vi "Close DO Ref.vi"(8 "error in (no error)":errorcluster, 11 "PXI 6515 in":refnum<class "PXI 6515.lvclass">) -> (0 "error out":errorcluster, 3 "PXI 6515 out":refnum<class "PXI 6515.lvclass">)   [LabVIEW 2016, in "DAQ IO.lvlib" / "PXI 6515.lvclass"]
uses:
  PXI 6515.lvclass
  PXI 6515.lvclass/PXI 6515.ctl
  <vilib>/DAQmx/write.llb/DAQmx Write (Digital Bool 1Line 1Point).vi
  <vilib>/DAQmx/miscellaneous.llb/DAQmx Fill In Error Info.vi
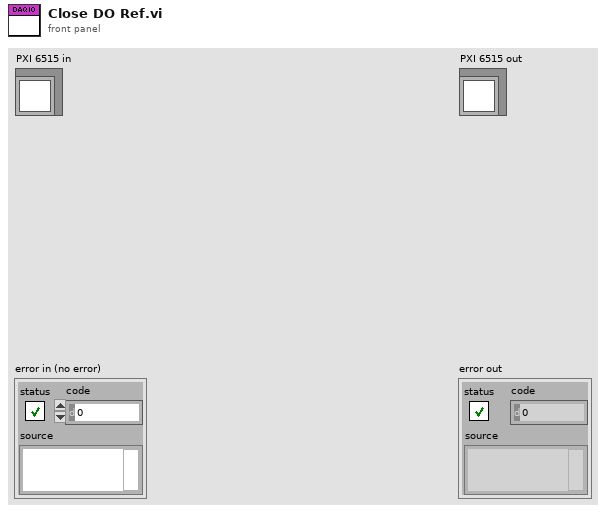
[diagram p1: front panel]
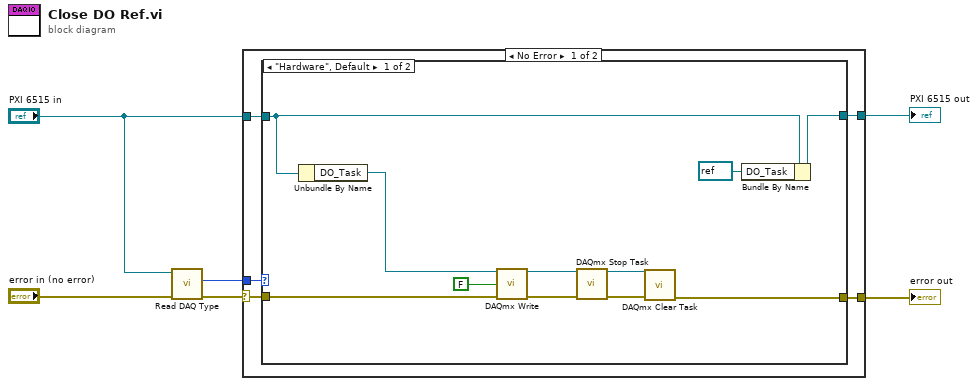
[diagram p0: block diagram]
diagram:
  n1 = call-dynamic "Read DAQ Type.vi"("error in (no error)"="error in (no error)", "PXI 6515 in"="PXI 6515 in") -> ("error out"=w5:errorcluster, "DAQ Type"=w4:enum16{"Hardware", "Simulation"})  [unwired: 7 in, 1 out]
  n2 = case shown="No Error" w5 {
    selector: w5 -> [w11 w25]
    tunnel: w4 -> [w10 _]
    tunnel: "PXI 6515 in" -> [w9 w26]
    tunnel: [w8 w25] -> w2
    tunnel: [w7 w26] -> w1
    frame No Error {
      n3 = case shown="\"Hardware\", Default" w10 {
        tunnel: w11 -> [w22 w23]
        tunnel: w9 -> [w20 w24]
        tunnel: [w21 w23] -> w8
        tunnel: [w19 w24] -> w7
        frame "Hardware", Default {
          n4 = Unbundle By Name(w20) -> ("DO_Task"=w13:refnum<k21>)
          n5 = call-poly <vilib>:"DAQmx Write.vi"("task/channels in"=w13, "data"=FALSE, "error in"=w22) -> ("task out"=w15:refnum<k21>, "error out"=w17:errorcluster)  [unwired: 10 in, 1 out]
          n6 = call <vilib>:"DAQmx Stop Task.vi"("task/channels in"=w15, "error in"=w17) -> ("task out"=w14:refnum<k21>, "error out"=w16:errorcluster)  [unwired: 12 in]
          n7 = call <vilib>:"DAQmx Clear Task.vi"("task in"=w14, "error in"=w16) -> ("error out"=w21:errorcluster)  [unwired: 13 in]
          n8 = Bundle By Name(cluster=w20, "DO_Task"=refnum<k21> refnum) -> (w19:refnum<class "PXI 6515.lvclass">)
        }
        frame "Simulation" {
        }
      }
    }
    frame Error {
    }
  }
  "error out" <- w2
  "PXI 6515 out" <- w1
